vi "ReadMutationHistory.vi"(8 "error in (no error)":errorcluster, 11 "LVClass path":path) -> (0 "error out":errorcluster, 1 "BlueSerializableVersion found?":bool, 2 "BlueSerializableVersion":u16, 3 "Mutation History":T1 {"LabVIEW Version" format="%.0x"})   [LabVIEW 2019, in "MutationHistoryGUI.lvlib"]
uses:
  MutationHistoryGUI.lvlib
  <vilib>/Utility/EditLVLibs/LVClass/Mutation History.ctl
  <vilib>/Utility/EditLVLibs/LVClass/Mutation Record.ctl
  <vilib>/Utility/EditLVLibs/LibVersion.ctl
  <resource>/Framework/Providers/BlueSerializationProviderShared/UserCommentToVersion.vi
  <vilib>/Utility/EditLVLibs/Edit LVLibs.lvlib
  <resource>/Framework/Providers/BlueSerializationProviderShared/BlueSerializationProviderShared.lvlib
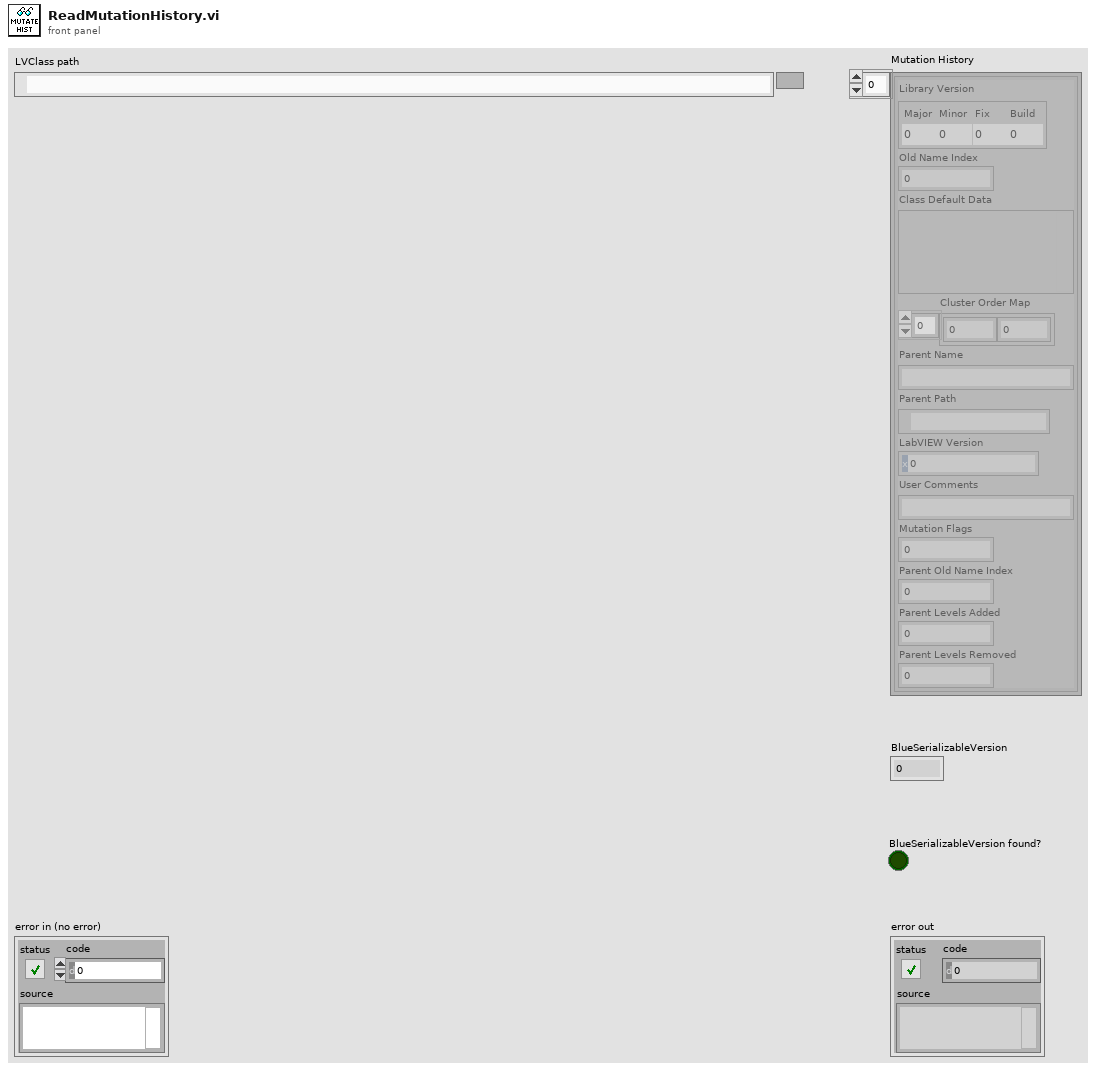
[diagram p1: front panel]
types:
  T1 = typedef "Edit LVLibs.lvlib/Mutation History.ctl" = T2[]
  T2 = typedef "Edit LVLibs.lvlib/Mutation Record.ctl" = cluster{"Library Version":T3, "Old Name Index":u8, "Class Default Data":variant, "Cluster Order Map":u32[], "Parent Name":string, "Parent Path":path, "LabVIEW Version":u32, "User Comments":string, "Mutation Flags":u8, "Parent Old Name Index":u8, "Parent Levels Added":u16, "Parent Levels Removed":u16}
  T3 = typedef "Edit LVLibs.lvlib/LibVersion.ctl" = cluster{"Major":u16, "Minor":u16, "Fix":u16, "Build":u16}
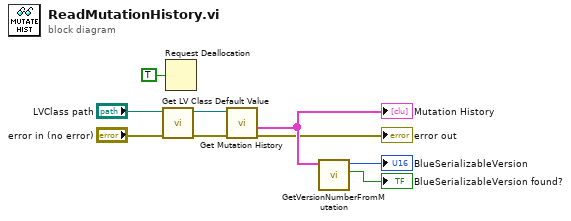
[diagram p0: block diagram]
diagram:
  n1 = call <vilib>:"Get LV Class Default Value.vi"("error in (no error)"="error in (no error)", "class path"="LVClass path") -> ("error out"=w4:errorcluster, "object"=w5:refnum<class>)  [unwired: 8 in]
  n2 = Request Deallocation(TRUE ("flag")) -> ()
  n3 = call <vilib>:"Get Mutation History.vi"("error in"=w4, "Input object"=w5) -> ("error out"=→"error out":errorcluster, "Mutation History"=w6:T1)  [unwired: 6 in]
  "Mutation History" <- w6
  n4 = call <resource>:"GetVersionNumberFromMutation.vi"("Mutation History"=w6) -> ("BlueSerializableVersion found?"=→"BlueSerializableVersion found?":bool, "BlueSerializableVersion"=→"BlueSerializableVersion":u16)  [unwired: 9 in]
